vi "Read Data Storage Data.vi"(0 "Device ID (0)":i32, 5 "Read Req":T4, 11 "error in (no error)":errorcluster) -> (4 "Device ID out":i32, 6 "Storage Data":u32[](array[numeric]), 8 "Storage Rsp":T1, 14 "Storage Info":T3, 15 "error out":errorcluster)   [LabVIEW 8.6, in "Keyence LJ-V7000.lvlib"]
doc: "Storage data will be acquired if \"storage target\" is set to \"OUT value\". Data acquisition is possible even during storage.\n\nIf there is no data stored, 0 will be output to \"<B>Read Data Cnt</B>\" of <B>Storage Rsp</B>.\nIf there is no stored data specified with \"<B>Start Data No</B>\" of <B>Read Req</B>, one piece of the latest data stored will be returned."
uses:
  Keyence LJ-V7000.lvlib
  constant/Driver VI No.ctl
  Clusters/Storage Info.ctl
  Clusters/Time.ctl
  Clusters/Read Storage Rsp.ctl
  Private/vi/Low Level/Make DLL Param(Read Storage Rsp).vi
  Private/vi/Low Level/Make VI Param(Read Storage Rsp).vi
  Clusters/Read Storage Req.ctl
panel:
  # "(c) 2012 KEYENCE CORPORATION.  ALL RIGHTS RESERVED."
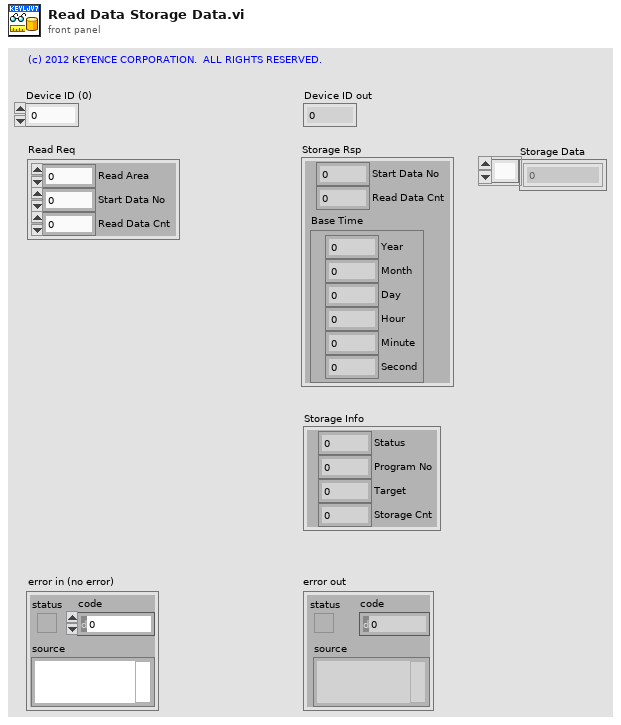
[diagram p1: front panel]
types:
  T1 = typedef "Keyence LJ-V7000.lvlib/Read Storage Rsp.ctl" = cluster{"Start Data No":u32, "Read Data Cnt":u32, "Base Time":T2}
  T2 = typedef "Keyence LJ-V7000.lvlib/Time.ctl" = cluster{"Year":u8, "Month":u8, "Day":u8, "Hour":u8, "Minute":u8, "Second":u8}
  T3 = typedef "Keyence LJ-V7000.lvlib/Storage Info.ctl" = cluster{"Status":u8, "Program No":u8, "Target":u8, "Storage Cnt":u32}
  T4 = typedef "Keyence LJ-V7000.lvlib/Read Storage Req.ctl" = cluster{"Read Area":u32, "Start Data No":u32, "Read Data Cnt":u32}
  T5 = typedef "Keyence LJ-V7000.lvlib/Driver VI No.ctl" = enum16{"Initialize", "Close", "Reboot Controller", "Return to Factory State", "Get System Error", "Clear System Error", "Trigger", "Start Batch Measurements", "Stop Batch Measurements", "Auto Zero", "Timing", "Reset", "Clear Memory", "Set Setting", "Get Setting", "Initialize Setting", "Reflect Setting", "Update Write Settings Area", "Check Status of Saving to Save Area", "Set Time", "Get Time", "Change Program", "Read Active Program Number", "Read Measurement Data", "Read Profiles(for High-Speed Mode)", "Read Batch Profiles(for High-Speed Mode)", "Read Profiles(for Advanced Mode)", "Read Batch Profiles(for Advanced Mode)", "Start Storage", "Stop Storage", "Read Storage Status", "Read Data Storage Data", "Read Profile Storage Data", "Read Batch Profile Storage Data", "Start High-Speed Data Communication", "Stop High-Speed Data Communication", "Read Profiles(for High-Speed Communication)"}
  T6 = cluster{"reserved":u8, "reserved":u8, "reserved":u8, "reserved":u8, "Read Area":u32, "Start Data No":u32, "Read Data Cnt":u32}
  T7 = cluster{"Status":u8, "Program No":u8, "Target":u8, "reserved":u8, "reserved":u8, "reserved":u8, "reserved":u8, "reserved":u8, "Storage Cnt":u32}
  T8 = cluster{"Start Data No":u32, "Read Data Cnt":u32, "pTime":cluster{"Year":u8, "Month":u8, "Day":u8, "Hour":u8, "Minute":u8, "Second":u8, "reserved":u8, "reserved":u8}}
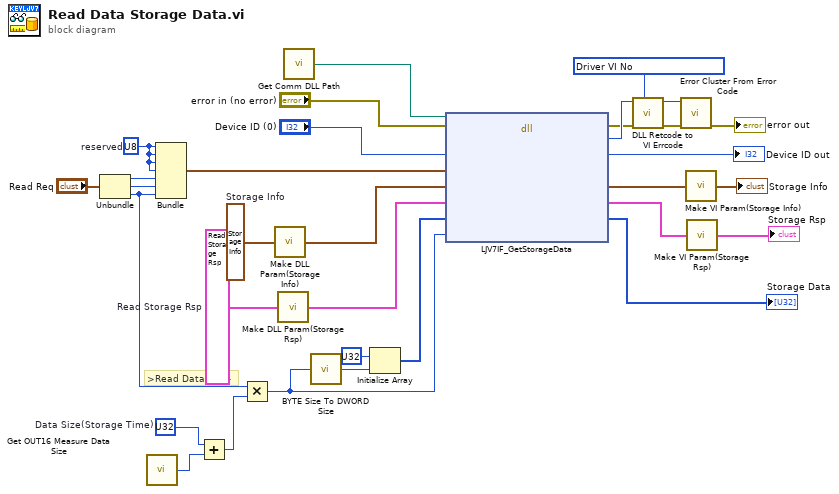
[diagram p0: block diagram]
diagram:
  w14 = u32 ?  # Data Size(Storage Time)
  w18 = T1 ?  # Read Storage Rsp
  w22 = T3 ?  # Storage Info
  w24 = u8 ?  # reserved
  # ">Read Data Cnt>"
  n1 = Unbundle("Read Req") -> ("Read Area"=w26:u32, "Start Data No"=w25:u32, "Read Data Cnt"=w12:u32)
  n2 = call "Get OUT16 Measure Data Size.vi"() -> ("OUT16 Measure Data Size"=w11:u32)  [unwired: 1 in]
  n3 = Bundle("reserved"=w24, "reserved"=w24, "reserved"=w24, "reserved"=w24, "Read Area"=w26, "Start Data No"=w25, "Read Data Cnt"=w12) -> (w23:T6)  [unwired: 1 in]
  n4 = Add(x=w14, y=w11) -> (x+y=w13:u32)
  n5 = Multiply(x=w12, y=w13) -> (x*y=w7:u32)
  n6 = call "Make DLL Param(Storage Info).vi"("Storage Info"=w22) -> ("pStorageInfo"=w21:T7)
  n7 = call-poly "Make DLL Param(Storage Rsp).vi"("Read Storage Rsp"=w18) -> ("pRsp"=w17:T8)
  n8 = call "Get Comm DLL Path.vi"() -> ("Comm DLL Path"=w30:path)  [unwired: 1 in]
  n9 = call "BYTE Size To DWORD Size.vi"("BYTE Size"=w7) -> ("DWORD Size"=w9:u32)
  n10 = Initialize Array(u32 ?, w9) -> (w8:u32[])
  n11 = dll-call lib="C:/Program Files/National Instruments/LabVIEW 2011/instr.lib/Keyence LJ-V7000/LJV7_IF.*" fn="LJV7IF_GetStorageData"(path in=w30, error in="error in (no error)", "lDeviceId"="Device ID (0)", "pReq"=w23, "pStorageInfo"=w21, "pRsp"=w17, "pdwData"=w8, "dwDataSize"=w7) -> (error out=w3:errorcluster, "lRetCode"=w4:i32, "lDeviceId"=→"Device ID out":i32, "pStorageInfo"=w19:T7, "pRsp"=w16:T8, "pdwData"=→"Storage Data":u32[])  [unwired: 3 in, 1 out]
  n12 = call "DLL Retcode to VI Errcode.vi"("Driver VI No"=T5 ?, "error in (no error)"=w3, "DLL Return Code"=w4) -> ("error out"=w6:errorcluster, "VI Error Code"=w5:i32)  [unwired: 7 in]
  n13 = call <vilib>:"Error Cluster From Error Code.vi"("error in (no error)"=w6, "error code (0)"=w5) -> ("error out"=→"error out":errorcluster)  [unwired: 7 in]
  n14 = call "Make VI Param(Storage Info).vi"("pStorageInfo"=w19) -> ("Storage Info"=→"Storage Info":T3)
  n15 = call-poly "Make VI Param(Storage Rsp).vi"("pRsp"=w16) -> ("Read Storage Rsp"=→"Storage Rsp":T1)
